vi "BlockDiagram_SetDefaults.vi"(7 "PythonConverter in":refnum<class "PythonBDConverter.lvclass">, 8 "error in":errorcluster, 11 "VI Interpreter in":refnum<class "VI Interpreter.lvclass">) -> (0 "error out":errorcluster, 3 "VI Interpreter out":refnum<class "VI Interpreter.lvclass">, 4 "set_defaults":string, 5 "PythonConverter out":refnum<class "PythonBDConverter.lvclass">)   [LabVIEW 2014, in "PythonBDConverter.lvclass"]
uses:
  PythonBDConverter.lvclass
  VI Interpreter/Classes/VI Interpreter/VI Interpreter.lvclass
  Parsing/ClassTypeTD.ctl
  VI Interpreter/Classes/ControlTerminal/ControlTerminal.lvclass
  VI Interpreter/Classes/TopLevelDiagram/TopLevelDiagram.lvclass
  Parsing/Python Functions.lvlib
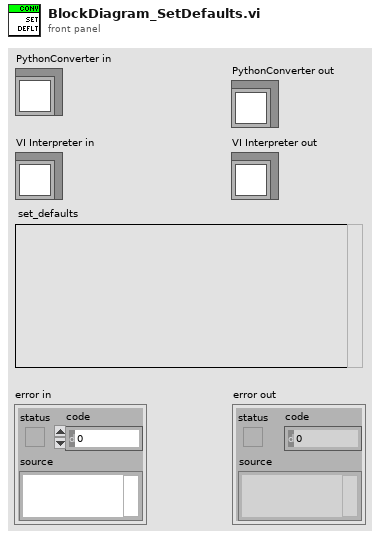
[diagram p1: front panel]
types:
  T1 = typedef "Python Functions.lvlib/ClassTypeTD.ctl" = enum16{"class", "function"}
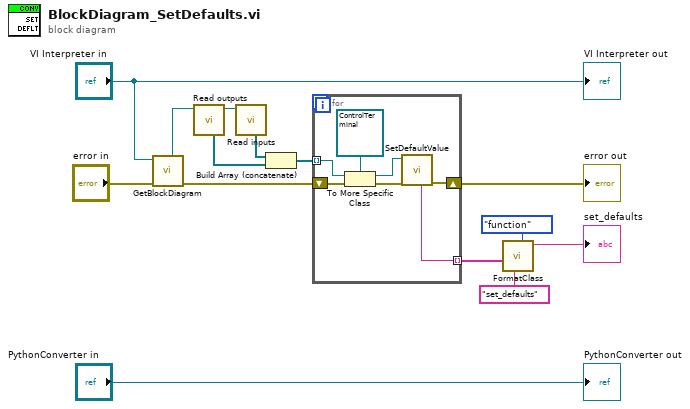
[diagram p0: block diagram]
diagram:
  n1 = call "GetBlockDiagram.vi"("error in"="error in", "VI Interpreter in"="VI Interpreter in") -> ("error out"=w9:errorcluster, "TopLevelDiagram"=w3:refnum<class "TopLevelDiagram.lvclass">)  [unwired: 5 in, 1 out]
  n2 = call-dynamic "Read outputs.vi"("Diagram in"=w3) -> ("Diagram out"=w4:refnum<class "TopLevelDiagram.lvclass">, "outputs"=w1:refnum<class "Terminal.lvclass">[])  [unwired: 7 in]
  n3 = call-dynamic "Read inputs.vi"("Diagram in"=w4) -> ("inputs"=w10:refnum<class "Terminal.lvclass">[])  [unwired: 7 in, 1 out]
  n4 = Build Array (concatenate)(w10, w1) -> (w2:refnum<class "Terminal.lvclass">[])
  n5 = for {
    tunnel: w2 -> [w19] mode=indexing
    shift-right: [w16] -> w8
    shift-left: w9 -> [w21]
    tunnel: [w15] -> w11 mode=indexing
    n6 = To More Specific Class(target class=refnum<class "ControlTerminal.lvclass"> refnum ("Control Terminal in"), reference=w19, error in=w21) -> (specific class reference=w17:refnum<class "ControlTerminal.lvclass">, error out=w18:errorcluster)
    n7 = call "SetDefaultValue.vi"("error in"=w18, "Control Terminal in"=w17) -> ("error out"=w16:errorcluster, "default"=w15:string)  [unwired: 5 in, 1 out]
  }
  "error out" <- w8
  n8 = call "FormatClass.vi"("type"=ClassTypeTD."function", "name"="set_defaults", "body"=w11) -> ("python"=→"set_defaults":string)  [unwired: 8 in]
  "PythonConverter out" <- "PythonConverter in"
  "VI Interpreter out" <- "VI Interpreter in"
